vi "APT move once.vi"(0 "reference":refnum<k7>, 1 "scale":sgl, 2 "error in (no error)":errorcluster, 3 "direction(0)":i32, 4 "state (2)":i32, 5 "A0":sgl) -> (14 "reference out":refnum<k7>, 15 "error out":errorcluster, 17 "x .and. y?":bool, 19 "GetPosition_Position":sgl)   [LabVIEW 2023]
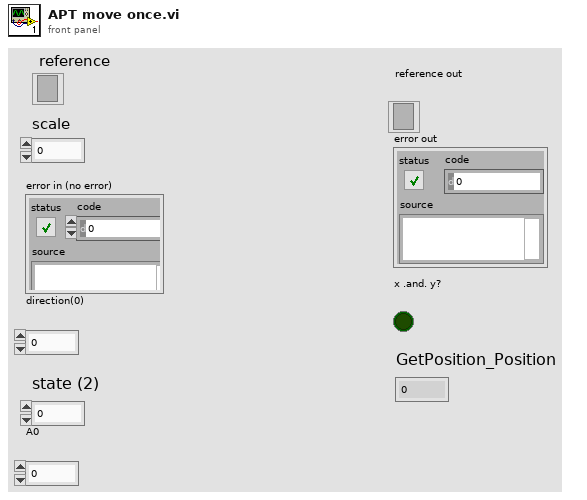
[diagram p1: front panel]
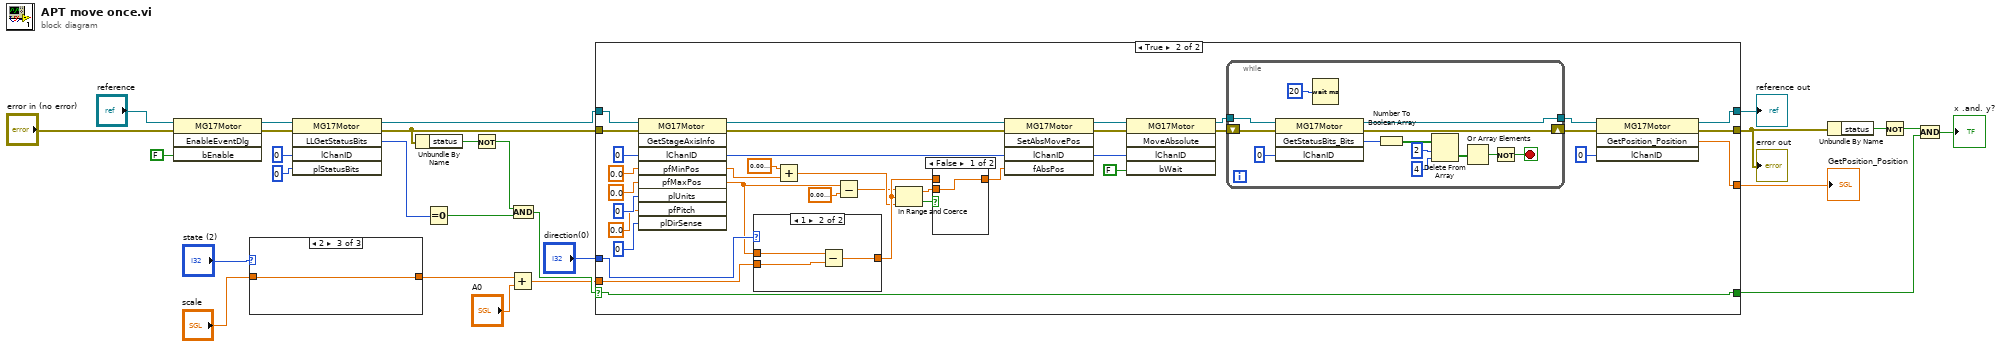
[diagram p0: block diagram]
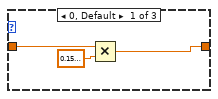
[diagram p2: hidden frame]
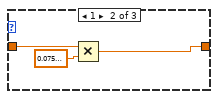
[diagram p3: hidden frame]
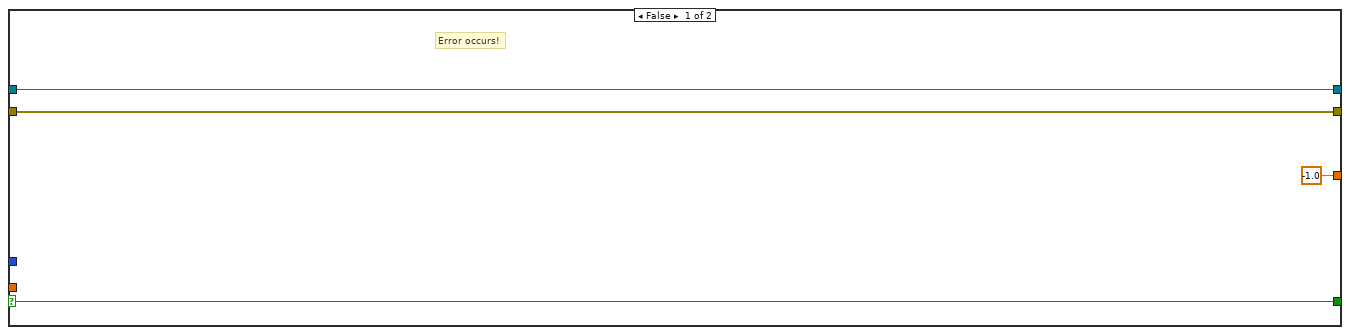
[diagram p4: hidden frame]
diagram:
  n1 = invoke class="MG17Motor" method="EnableEventDlg"(reference="reference", error in="error in (no error)", "bEnable"=FALSE) -> (reference out=w5:refnum<k7>, error out=w4:errorcluster)  [unwired: 1 in, 2 out]
  n2 = case shown="2" "state (2)" {
    tunnel: [w29 w31 w34] -> w12
    tunnel: "scale" -> [w28 w32 w34]
    frame 0, Default {
      n3 = Multiply(x=w28, y=sgl 0.15) -> (x*y=w29:sgl)
    }
    frame 1 {
      n4 = Multiply(x=w32, y=sgl 0.075) -> (x*y=w31:sgl)
    }
    frame 2 {
    }
  }
  n5 = invoke class="MG17Motor" method="LLGetStatusBits"(reference=w5, error in=w4, "lChanID"=0, "plStatusBits"=0) -> (reference out=w24:refnum<k7>, error out=w22:errorcluster, "LLGetStatusBits"=w25:i32)  [unwired: 1 in, 2 out]
  n6 = Unbundle By Name(w22) -> ("status"=w19:bool)
  n7 = Equal To 0?(x=w25) -> (x = 0?=w21:bool)
  n8 = Not(x=w19) -> (.not. x?=w18:bool)
  n9 = Add(x=w12, y="A0") -> (x+y=w2:sgl)
  n10 = And(x=w18, y=w21) -> (x .and. y?=w20:bool)
  n11 = case shown="True" w20 {
    selector: w20 -> [w37 w71]
    tunnel: w24 -> [w35 w68]
    tunnel: w22 -> [w38 w67]
    tunnel: [w38 w41] -> w9
    tunnel: [w37 w71] -> w23
    tunnel: "direction(0)" -> [_ w70]
    tunnel: w2 -> [_ w69]
    tunnel: [sgl -1.0 ("GetPosition_Position") w39] -> w10
    tunnel: [w35 w44] -> w8
    frame False {
      # "Error occurs!"
    }
    frame True {
      n12 = invoke class="MG17Motor" method="GetStageAxisInfo"(reference=w68, error in=w67, "lChanID"=0, "pfMinPos"=sgl 0.0, "pfMaxPos"=sgl 0.0, "plUnits"=0, "pfPitch"=sgl 0.0, "plDirSense"=0) -> (reference out=w66:refnum<k7>, error out=w65:errorcluster, "lChanID"=w63:i32, "pfMinPos"=w56:sgl, "pfMaxPos"=w46:sgl)  [unwired: 1 in, 4 out]
      n13 = case shown="1" w70 {
        tunnel: [w90 w92] -> w54
        tunnel: w69 -> [w90 w93]
        tunnel: w46 -> [_ w91]
        frame 0, Default {
        }
        frame 1 {
          n14 = Subtract(x=w91, y=w93) -> (x-y=w92:sgl)
        }
      }
      n15 = Add(x=sgl 0.01, y=w56) -> (x+y=w50:sgl)
      n16 = Subtract(x=w46, y=sgl 0.01) -> (x-y=w49:sgl)
      n17 = In Range and Coerce(upper limit=w49, x=w54, lower limit=w50) -> (coerced(x)=w53:sgl, In Range?=w55:bool)
      n18 = case shown="False" w55 {
        tunnel: [w88 w89] -> w40
        tunnel: w54 -> [_ w89]
        tunnel: w53 -> [w88 _]
        frame False {
        }
        frame True {
        }
      }
      n19 = invoke class="MG17Motor" method="SetAbsMovePos"(reference=w66, error in=w65, "lChanID"=w63, "fAbsPos"=w40) -> (reference out=w73:refnum<k7>, error out=w72:errorcluster, "lChanID"=w62:i32)  [unwired: 1 in, 2 out]
      n20 = invoke class="MG17Motor" method="MoveAbsolute"(reference=w73, error in=w72, "lChanID"=w62, "bWait"=FALSE) -> (reference out=w51:refnum<k7>, error out=w52:errorcluster)  [unwired: 1 in, 3 out]
      n21 = while {
        shift-right: [w86] -> w42
        shift-left: w52 -> [w87]
        tunnel: w51 -> [w82]
        tunnel: [w80] -> w48
        stop <- w81 stop-if-true
        n22 = invoke class="MG17Motor" method="GetStatusBits_Bits"(reference=w82, error in=w87, "lChanID"=0) -> (reference out=w80:refnum<k7>, error out=w86:errorcluster, "GetStatusBits_Bits"=w83:i32)  [unwired: 1 in, 1 out]
        n23 = Wait (ms)(milliseconds to wait=u32 20) -> ()  [unwired: 1 out]
        n24 = Number To Boolean Array(number=w83) -> (Boolean array=w78:bool[])
        n25 = Delete From Array "Delete From Array"(array=w78, length=2 ("index"), index=4) -> (deleted portion=w76:bool[])  [unwired: 1 out]
        n26 = Or Array Elements(Boolean array=w76) -> (logical OR=w75:bool)
        n27 = Not(x=w75) -> (.not. x?=w81:bool)
      }
      n28 = invoke class="MG17Motor" method="GetPosition_Position"(reference=w48, error in=w42, "lChanID"=0) -> (reference out=w44:refnum<k7>, error out=w41:errorcluster, "GetPosition_Position"=w39:sgl)  [unwired: 1 in, 1 out]
    }
  }
  "GetPosition_Position" <- w10
  "reference out" <- w8
  "error out" <- w9
  n29 = Unbundle By Name(w9) -> ("status"=w17:bool)
  n30 = Not(x=w17) -> (.not. x?=w16:bool)
  n31 = And(x=w16, y=w23) -> (x .and. y?=→"x .and. y?":bool)
